vi "DatLog.vi"() -> ()   [LabVIEW 2020]
uses:
  <vilib>/Utility/error.llb/DialogType.ctl
panel:
  in  "LogFile":path
  out "error out":errorcluster
  in  "error in":errorcluster
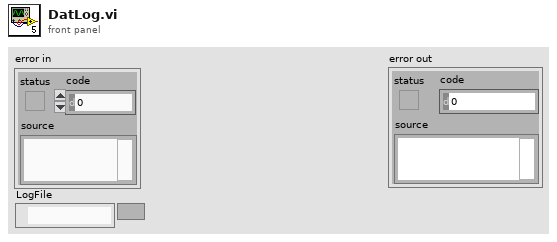
[diagram p1: front panel]
types:
  T1 = typedef "DialogType.ctl" = u16
  T2 = cluster{"Time Stamp":timestamp, "error":errorcluster}
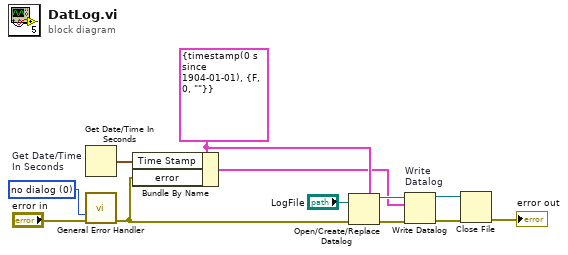
[diagram p0: block diagram]
diagram:
  w5 = T1 0 items=["no dialog", "OK message", "continue or stop message", "OK message + warnings", "continue/stop + warnings"] ("type of dialog (OK msg:1)")
  w8 = T2 {"Time Stamp"=timestamp(0 s since 1904-01-01), "error"={"status"=FALSE, "code"=0, "source"=""}} ("record type")
  n1 = Get Date/Time In Seconds "Get Date/Time\nIn Seconds"() -> (seconds since 1Jan1904=w7:timestamp)
  n2 = call <vilib>:"General Error Handler.vi"("type of dialog (OK msg:1)"=w5, "error in (no error)"="error in") -> ("error out"=w3:errorcluster)  [unwired: 9 in, 4 out]
  n3 = Bundle By Name(cluster=w8, "Time Stamp"=w7, "error"=w3) -> (w6:T2)
  n4 = Open/Create/Replace Datalog(5:w8, 8:w3, 11:"LogFile") -> (0:w10:errorcluster, 3:w12:refnum<k1>)  [unwired: 3 in, 1 out]
  n5 = Write Datalog "Write\nDatalog"(4:w10, 6:w6, 7:w12) -> (0:w9:errorcluster, 3:w11:refnum<k1>)
  n6 = Close File(refnum=w11, error in=w9) -> (error out=→"error out":errorcluster)  [unwired: 1 out]
